vi "Create and Destroy Session.vi"(8 "error in (no error)":errorcluster) -> (0 "error out":errorcluster)   [LabVIEW 2020]
uses:
  G-Embedded-Python-Interpreter-Toolkit/Merge Call Library Errors.vi
  <vilib>/addons/_JKI Toolkits/Caraya/classes/Assert/Assert Error.vi
  <vilib>/addons/_JKI Toolkits/Caraya/classes/Assert/Assert Not Error.vi
  G-Embedded-Python-Interpreter-Toolkit/G-Embedded-Python-Interpreter-Toolkit.lvlib
  <vilib>/addons/_JKI Toolkits/Caraya/classes/Assert/Assert.lvclass
  <vilib>/addons/_JKI Toolkits/Caraya/classes/Test/Test.lvclass
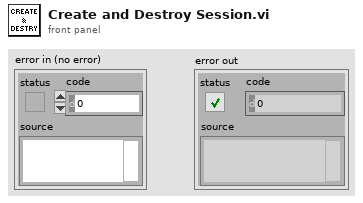
[diagram p1: front panel]
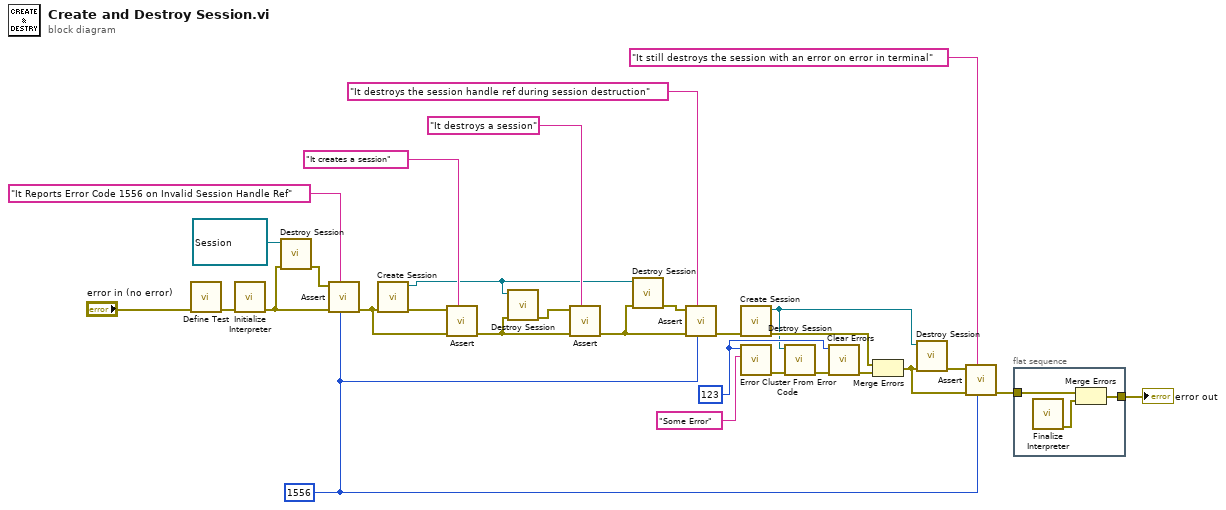
[diagram p0: block diagram]
diagram:
  w11 = 123 ("error code (0)")
  w1 = 1556 ("error code (1)")
  n1 = call <vilib>:"Define Test.vi"("error in (no error)"="error in (no error)") -> ("error out"=w30:errorcluster)  [unwired: 10 in]
  n2 = call "Initialize Interpreter.vi"("error in (no error)"=w30) -> ("error out"=w22:errorcluster)  [unwired: 9 in, 1 out]
  n3 = call "Destroy Session.vi"("error in (no error)"=w22, "Session Handle"=refnum<data-value> refnum) -> ("error out"=w23:errorcluster)  [unwired: 9 in]
  n4 = call-poly <vilib>:"Assert.vi"("error code (1)"=w1, "Label"="It Reports Error Code 1556 on Invalid Session Handle Ref", "error in (no error)"=w22, "Error?"=w23) -> ("error out"=w20:errorcluster)  [unwired: 7 in]
  n5 = call "Create Session.vi"("error in (no error)"=w20) -> ("error out"=w27:errorcluster, "Session Handle"=w18:refnum<data-value>)  [unwired: 9 in]
  n6 = call-poly <vilib>:"Assert.vi"("Label"="It creates a session", "error in (no error)"=w20, "Not Error?"=w27) -> ("error out"=w25:errorcluster)  [unwired: 8 in]
  n7 = call "Destroy Session.vi"("error in (no error)"=w25, "Session Handle"=w18) -> ("error out"=w26:errorcluster)  [unwired: 9 in]
  n8 = call-poly <vilib>:"Assert.vi"("Label"="It destroys a session", "error in (no error)"=w25, "Not Error?"=w26) -> ("error out"=w16:errorcluster)  [unwired: 8 in]
  n9 = call "Destroy Session.vi"("error in (no error)"=w16, "Session Handle"=w18) -> ("error out"=w17:errorcluster)  [unwired: 9 in]
  n10 = call-poly <vilib>:"Assert.vi"("error code (1)"=w1, "Label"="It destroys the session handle ref during session destruction", "error in (no error)"=w16, "Error?"=w17) -> ("error out"=w14:errorcluster)  [unwired: 7 in]
  n11 = call "Create Session.vi"("error in (no error)"=w14) -> ("error out"=w8:errorcluster, "Session Handle"=w7:refnum<data-value>)  [unwired: 9 in]
  n12 = call <vilib>:"Error Cluster From Error Code.vi"("error message (\"\")"="Some Error" ("error message (\"\")"), "error code (0)"=w11) -> ("error out"=w12:errorcluster)  [unwired: 7 in]
  n13 = call "Destroy Session.vi"("error in (no error)"=w12, "Session Handle"=w7) -> ("error out"=w13:errorcluster)  [unwired: 9 in]
  n14 = call <vilib>:"Clear Errors.vi"("error in (no error)"=w13, "specific error code to clear (0: all)"=w11) -> ("error out"=w9:errorcluster)  [unwired: 4 in, 1 out]
  n15 = Merge Errors(w8, w9) -> (w5:errorcluster)
  n16 = call "Destroy Session.vi"("error in (no error)"=w5, "Session Handle"=w7) -> ("error out"=w6:errorcluster)  [unwired: 9 in]
  n17 = call-poly <vilib>:"Assert.vi"("error code (1)"=w1, "Label"="It still destroys the session with an error on error in terminal", "error in (no error)"=w5, "Error?"=w6) -> ("error out"=w3:errorcluster)  [unwired: 7 in]
  n18 = flat-sequence {
    tunnel: w3 -> [w33]
    tunnel: [w31] -> w2
    frame #0 {
      n19 = call "Finalize Interpreter.vi"() -> ("error out"=w32:errorcluster)  [unwired: 11 in]
      n20 = Merge Errors(w33, w32) -> (w31:errorcluster)
    }
  }
  "error out" <- w2
